vi "FABR-Restore Defaults.vi"() -> (4 "Params":T1={"Format"=20, "Stimulus"={"Destination"="", "Rep rate (/sec)"=30.0, "Alternate Polarity"=FALSE, "Duration (ms)"=0.0, "Ramp (ms)"=16.0, "Fs (Hz)"=5.0, "Frame size (s)"=0.0}, "Sequence"={"Freq"={"Expression"="", "Skip"=80}, "Level"={"Start (dB)"=20, "Stop (dB)"=80, "Step (dB)"=5}, "Order"=enum."Interleaved"}, "Response"={"Gain"=1.0, "Averages"=0, "Window (ms)"=0.0, "Fs (Hz)"=25000.0, "Save raw"=FALSE}, "Reject"=0.0} {"Sequence"."Level"."Start (dB)" step=5; "Response"."Window (ms)" format="%.2f"}, 8 "Threshold Estimation":T6={"Tmin (ms)"=1.0, "Tmax (ms)"=6.0, "CC criterion"=0.35, "adjR2 criterion"=0.7}, 15 "error out":errorcluster)   [LabVIEW 2020]
uses:
  Typedefs/FABR-Parameters.ctl
  Typedefs/FABR-Stimulus.ctl
  Typedefs/FABR-Sequence.ctl
  Typedefs/FABR-Order.ctl
  Typedefs/FABR-Response.ctl
  Threshold Estimation VIs/ABR3-Threshold Estimation Parameters.ctl
  Typedefs/Legacy/FABR-Parameters V1.ctl
panel:
  in  "Default":T1={"Format"=-1, "Stimulus"={"Destination"="Right ear", "Rep rate (/sec)"=50.0, "Alternate Polarity"=FALSE, "Duration (ms)"=5.0, "Ramp (ms)"=0.5, "Fs (Hz)"=100000.0, "Frame size (s)"=1.0}, "Sequence"={"Freq"={"Expression"="4:0.5oct:48", "Skip"=1}, "Level"={"Start (dB)"=20, "Stop (dB)"=50, "Step (dB)"=5}, "Order"=enum."Interleaved"}, "Response"={"Gain"=10000.0, "Averages"=512, "Window (ms)"=8.5, "Fs (Hz)"=25000.0, "Save raw"=FALSE}, "Reject"=15.0} {"Sequence"."Level"."Start (dB)" step=5; "Response"."Window (ms)" format="%.2f"}
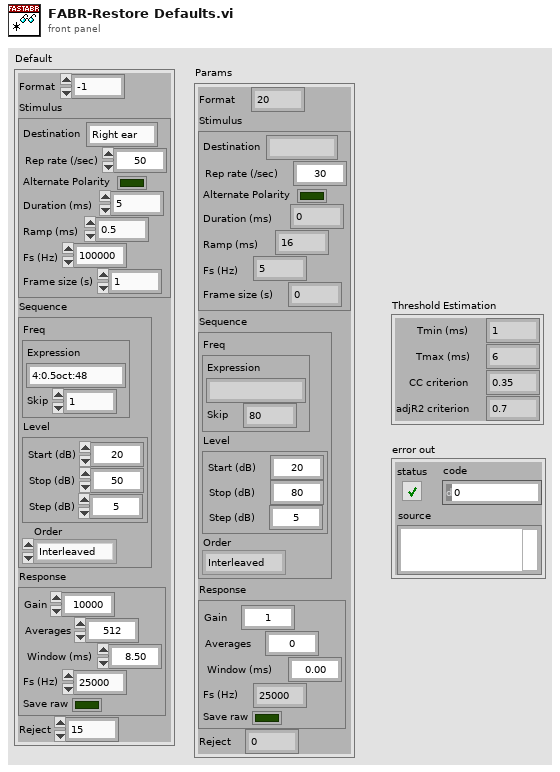
[diagram p1: front panel]
types:
  T1 = typedef "FABR-Parameters.ctl" = cluster{"Format":i32, "Stimulus":T2, "Sequence":T3, "Response":T5, "Reject":dbl}
  T2 = typedef "FABR-Stimulus.ctl" = cluster{"Destination":string, "Rep rate (/sec)":dbl, "Alternate Polarity":bool, "Duration (ms)":dbl, "Ramp (ms)":dbl, "Fs (Hz)":dbl, "Frame size (s)":dbl}
  T3 = typedef "FABR-Sequence.ctl" = cluster{"Freq":cluster{"Expression":string, "Skip":i32}, "Level":cluster{"Start (dB)":i32, "Stop (dB)":i32, "Step (dB)":i32}, "Order":T4}
  T4 = typedef "FABR-Order.ctl" = enum16{"Interleaved"}
  T5 = typedef "FABR-Response.ctl" = cluster{"Gain":dbl, "Averages":i32, "Window (ms)":sgl, "Fs (Hz)":dbl, "Save raw":bool}
  T6 = typedef "ABR3-Threshold Estimation Parameters.ctl" = cluster{"Tmin (ms)":dbl, "Tmax (ms)":dbl, "CC criterion":dbl, "adjR2 criterion":dbl}
  T7 = typedef "FABR-Parameters V1.ctl" = cluster{"Stimulus":T2, "Sequence":cluster{"Freq":cluster{"Start (kHz)":dbl, "Stop (kHz)":dbl, "Step (oct)":dbl, "Skip (oct)":dbl}, "Level":cluster{"Start (dB)":i32, "Stop (dB)":i32, "Step (dB)":i32}, "Order":T4}, "Response":T5, "Reject":dbl}
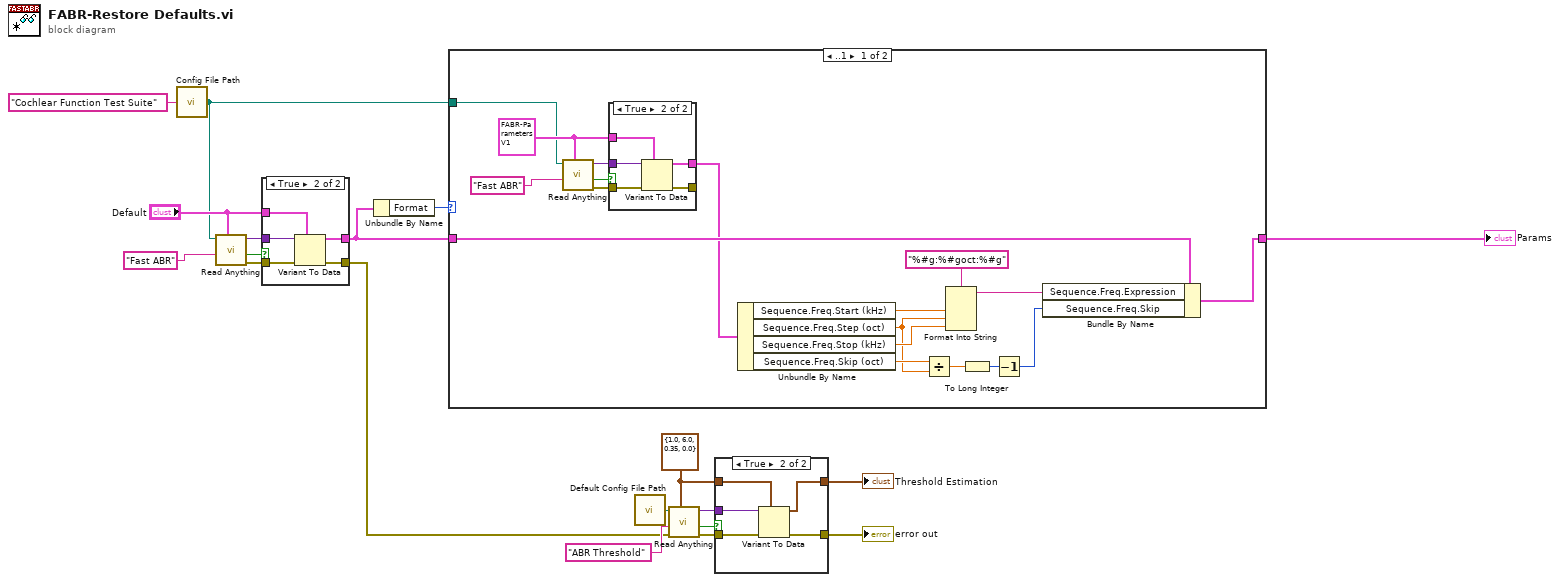
[diagram p0: block diagram]
diagram:
  w14 = T6 {"Tmin (ms)"=1.0, "Tmax (ms)"=6.0, "CC criterion"=0.35, "adjR2 criterion"=0.0} ("Threshold Estimation")
  n1 = call "Config File Path.vi"("AppName"="Cochlear Function Test Suite") -> ("Default config file name"=w2:path)
  n2 = call "Read Anything.vi"("Type of Anything"="Default", "Section Name (Name of \"Type of Anything\")"="Fast ABR" ("Section Name (Name of \"Type of Anything\")"), "Path (dialog)"=w2) -> ("Error Out"=w17:errorcluster, "Found?"=w6:bool, "Anything"=w19:variant)  [unwired: 6 in]
  n3 = case shown="True" w6 {
    tunnel: w19 -> [_ w26]
    tunnel: w17 -> [w20 w25]
    tunnel: [w21 w24] -> w3
    tunnel: [w20 w23] -> w11
    tunnel: "Default" -> [w21 w22]
    frame False {
    }
    frame True {
      n4 = Variant To Data(error in=w25, type=w22, Variant=w26) -> (data=w24:T1, error out=w23:errorcluster)
    }
  }
  n5 = Unbundle By Name(w3) -> ("Format"=w4:i32)
  n6 = case shown="..1" w4 {
    tunnel: w3 -> [w38 w52]
    tunnel: w2 -> [w39 _]
    tunnel: [w36 w52] -> w1
    frame ..1 {
      w40 = T7 {"Stimulus"={"Destination"="", "Rep rate (/sec)"=30.0, "Alternate Polarity"=FALSE, "Duration (ms)"=0.0, "Ramp (ms)"=16.0, "Fs (Hz)"=5.0, "Frame size (s)"=0.0}, "Sequence"={"Freq"={"Start (kHz)"=20.0, "Stop (kHz)"=80.0, "Step (oct)"=5.0, "Skip (oct)"=0.0}, "Level"={"Start (dB)"=20, "Stop (dB)"=80, "Step (dB)"=5}, "Order"=enum."Interleaved"}, "Response"={"Gain"=10000.0, "Averages"=512, "Window (ms)"=8.5, "Fs (Hz)"=25000.0, "Save raw"=FALSE}, "Reject"=0.0} ("Params")
      n7 = call "Read Anything.vi"("Type of Anything"=w40, "Section Name (Name of \"Type of Anything\")"="Fast ABR" ("Section Name (Name of \"Type of Anything\")"), "Path (dialog)"=w39) -> ("Error Out"=w42:errorcluster, "Found?"=w41:bool, "Anything"=w44:variant)  [unwired: 6 in]
      n8 = case shown="True" w41 {
        tunnel: w44 -> [_ w51]
        tunnel: w42 -> [w45 w50]
        tunnel: [w46 w49] -> w37
        tunnel: [w45 w48] -> _
        tunnel: w40 -> [w46 w47]
        frame False {
        }
        frame True {
          n9 = Variant To Data(error in=w50, type=w47, Variant=w51) -> (data=w49:T7, error out=w48:errorcluster)
        }
      }
      n10 = Unbundle By Name(w37) -> ("Sequence.Freq.Start (kHz)"=w34:dbl, "Sequence.Freq.Step (oct)"=w28:dbl, "Sequence.Freq.Stop (kHz)"=w32:dbl, "Sequence.Freq.Skip (oct)"=w31:dbl)
      n11 = Divide(x=w31, y=w28) -> (x/y=w30:dbl)
      n12 = Format Into String(format string="%#g:%#goct:%#g", w34, w28, w32) -> (resulting string=w33:string)  [unwired: 2 in, 1 out]
      n13 = To Long Integer(number=w30) -> (32bit integer=w29:i32)
      n14 = Decrement(x=w29) -> (x-1=w27:i32)
      n15 = Bundle By Name(cluster=w38, "Sequence.Freq.Expression"=w33, "Sequence.Freq.Skip"=w27) -> (w36:T1)
    }
    frame 2, Default {
    }
  }
  "Params" <- w1
  n16 = call "Default Config File Path.vi"() -> ("Default config file name"=w13:path)
  n17 = call "Read Anything.vi"("Type of Anything"=w14, "Error In"=w11, "Section Name (Name of \"Type of Anything\")"="ABR Threshold" ("Section Name (Name of \"Type of Anything\")"), "Path (dialog)"=w13) -> ("Error Out"=w8:errorcluster, "Found?"=w10:bool, "Anything"=w9:variant)  [unwired: 5 in]
  n18 = case shown="True" w10 {
    tunnel: w9 -> [_ w58]
    tunnel: w14 -> [w54 w57]
    tunnel: w8 -> [w53 w59]
    tunnel: [w54 w56] -> w15
    tunnel: [w53 w55] -> w16
    frame False {
    }
    frame True {
      n19 = Variant To Data(error in=w59, type=w57, Variant=w58) -> (data=w56:T6, error out=w55:errorcluster)
    }
  }
  "error out" <- w16
  "Threshold Estimation" <- w15
